vi "Comm visa old.vi"(8 "error in (no error)":errorcluster, 10 "send data":string, 11 "VISA resource name":refnum<visa-resource-name>) -> (0 "error out":errorcluster, 2 "read buffer":string, 3 "VISA resource name out":refnum<visa-resource-name>)   [LabVIEW 2014, in "AISAS motor.lvclass"]
uses:
  AISAS motor.lvclass
panel:
  out "bytes at port":u32
  out "i":i32
  out "return count":u32
  out "length":i32
  in  "response lenght (1B)":i32=1
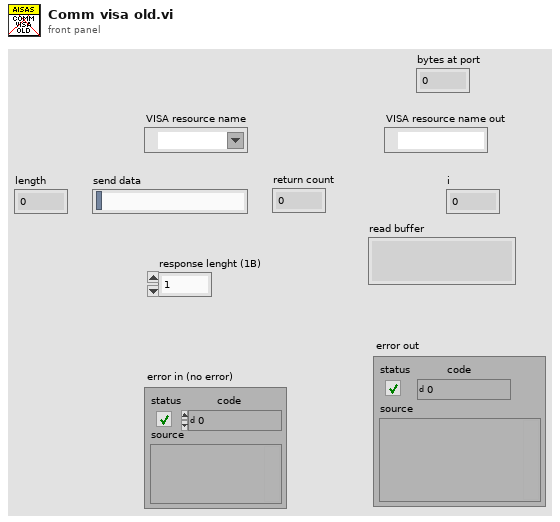
[diagram p1: front panel]
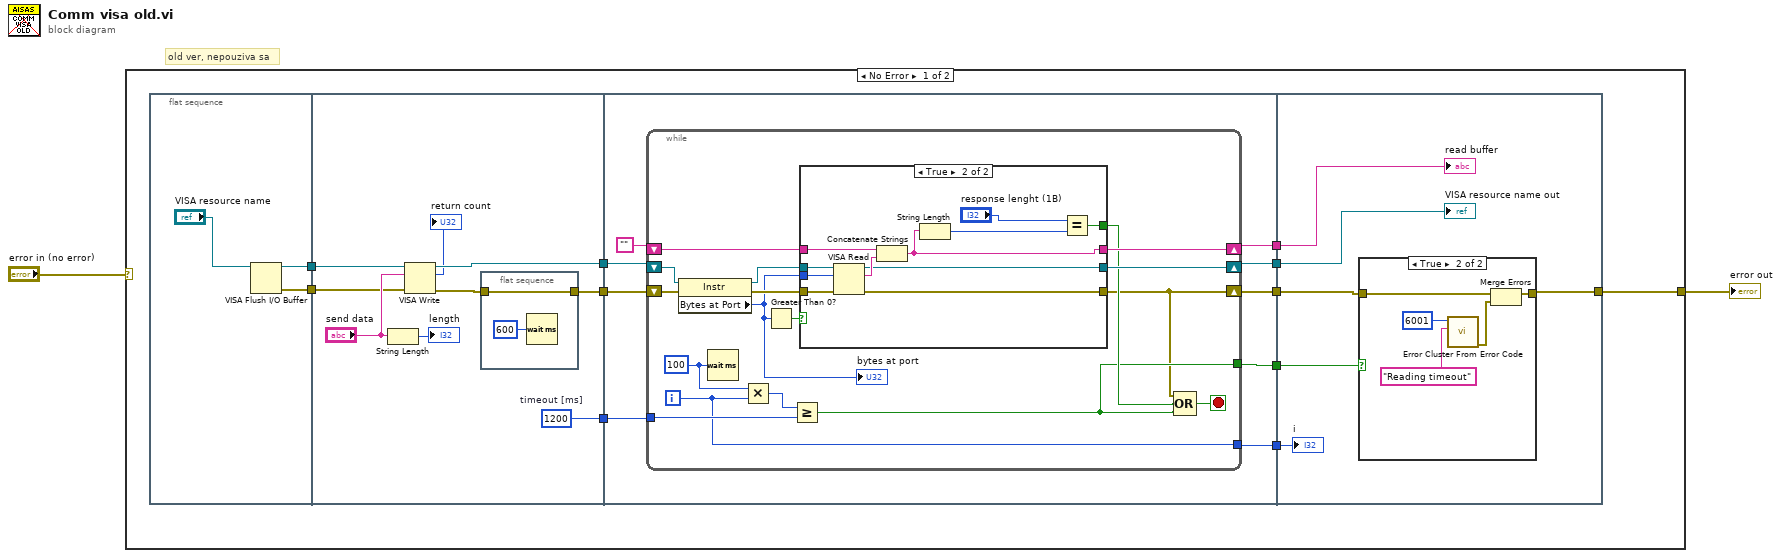
[diagram p0: block diagram]
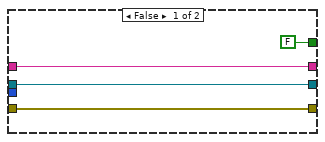
[diagram p2: hidden frame]
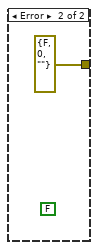
[diagram p4: hidden frame]
diagram:
  # "old ver, nepouziva sa"
  n1 = case shown="No Error" "error in (no error)" {
    tunnel: [w7 errorcluster {"status"=FALSE, "code"=0, "source"=""} ("error IO")] -> w1
    frame No Error {
      n2 = flat-sequence {
        tunnel: [w15] -> w5
        tunnel: [w14] -> w4
        tunnel: [w25] -> w13
        tunnel: [w18] -> w12
        tunnel: w5 -> [w21]
        tunnel: w4 -> [w20]
        tunnel: [w17] -> w3
        tunnel: w13 -> [w35]
        tunnel: w12 -> [w36]
        tunnel: [w34] -> w11
        tunnel: [w33] -> w10
        tunnel: [w32] -> w9
        tunnel: [w30] -> w8
        tunnel: [w29] -> w6
        tunnel: w3 -> [w28]
        tunnel: [w71] -> w7
        tunnel: w11 -> [w73]
        tunnel: w10 -> [w70]
        tunnel: w9 -> [w72]
        tunnel: w8 -> [w74]
        tunnel: w6 -> [w69]
        frame #0 {
          n3 = VISA Flush I/O Buffer(VISA resource name="VISA resource name") -> (VISA resource name out=w15:refnum<visa-resource-name>, error out=w14:errorcluster)  [unwired: 2 in]
        }
        frame #1 {
          w17 = u32 1200  # timeout [ms]
          n4 = String Length(string="send data") -> (length=→"length":i32)
          n5 = VISA Write(VISA resource name=w21, write buffer="send data", error in (no error)=w20) -> (VISA resource name out=w25:refnum<visa-resource-name>, return count=→"return count":u32, error out=w19:errorcluster)
          n6 = flat-sequence {
            tunnel: w19 -> [w27]
            tunnel: [w27] -> w18
            frame #0 {
              n7 = Wait (ms)(milliseconds to wait=u32 600) -> ()  [unwired: 1 out]
            }
          }
        }
        frame #2 {
          n8 = while {
            shift-right: [w50] -> w32
            shift-left: "" -> [w49]
            shift-right: [w48] -> w34
            shift-left: w35 -> [w47]
            shift-right: [w40] -> w33
            shift-left: w36 -> [w46]
            tunnel: w28 -> [w43]
            tunnel: [w41] -> w30
            tunnel: [w38] -> w29
            i -> [w38]
            stop <- w39 stop-if-true
            w45 = u32 100 ("milliseconds to wait")
            n9 = property class="Instr"(reference=w47, error in=w46) -> (reference out=w52:refnum<visa-resource-name>, error out=w53:errorcluster, "Bytes at Port"=w37:u32)
            "bytes at port" <- w37
            n10 = Wait (ms)(milliseconds to wait=w45) -> ()  [unwired: 1 out]
            n11 = Multiply(x=w45, y=w38) -> (x*y=w44:u32)
            n12 = Greater Than 0?(x=w37) -> (x > 0?=w51:bool)
            n13 = Greater Or Equal?(x=w44, y=w43) -> (x >= y?=w41:bool)
            n14 = case shown="True" w51 {
              tunnel: w53 -> [w55 w68]
              tunnel: w37 -> [_ w67]
              tunnel: w52 -> [w56 w66]
              tunnel: [w57 w61] -> w50
              tunnel: w49 -> [w57 w64]
              tunnel: [w56 w63] -> w48
              tunnel: [w55 w62] -> w40
              tunnel: [FALSE w60] -> w42
              frame False {
              }
              frame True {
                n15 = VISA Read(VISA resource name=w66, byte count=w67, error in (no error)=w68) -> (VISA resource name out=w63:refnum<visa-resource-name>, read buffer=w65:string, error out=w62:errorcluster)  [unwired: 1 out]
                n16 = Concatenate Strings(w64, w65) -> (w61:string)
                n17 = String Length(string=w61) -> (length=w59:i32)
                n18 = Equal?(x="response lenght (1B)", y=w59) -> (x = y?=w60:bool)
              }
            }
            n19 = Compound Arithmetic op=OR(w40, w42, w41) -> (w39:bool)
          }
        }
        frame #3 {
          n20 = case shown="True" w74 {
            tunnel: w70 -> [w75 w76]
            tunnel: [w75 w80] -> w71
            frame False {
            }
            frame True {
              n21 = call <vilib>:"Error Cluster From Error Code.vi"("error message (\"\")"="Reading timeout" ("error message (\"\")"), "error code (0)"=6001) -> ("error out"=w79:errorcluster)  [unwired: 7 in]
              n22 = Merge Errors(w76, w79) -> (w80:errorcluster)
            }
          }
          "read buffer" <- w72
          "VISA resource name out" <- w73
          "i" <- w69
        }
      }
    }
    frame Error {
      (unwired) FALSE
    }
  }
  "error out" <- w1
